vi "RX example.vi"() -> ()   [LabVIEW 2010]
uses:
  HackRF_Read_Complex.vi
  <vilib>/Analysis/NI_AALPro.lvlib
  <vilib>/Analysis/2dsp.llb/Complex FFT.vi
panel:
  out "Waveform Graph":dbl[](graph)
  in  "CarrierFreqHz":dbl(slide)=90658509.45494995 scale=86000000.0..110000000.0 scale format="%#_6p"
  in  "AMPEnable":bool
  in  "VGAGainDb":dbl=40.0 min=0.0 max=62.0 step=2.0
  in  "LNAGainDb":dbl=24.0 min=0.0 max=40.0 step=8.0
  in  "stop":bool
  in  "SampleFreqHz":dbl=4500000.0 format="%#_6p"
  in  "FilterBandwidthHz":dbl=3000000.0 format="%#_6p"
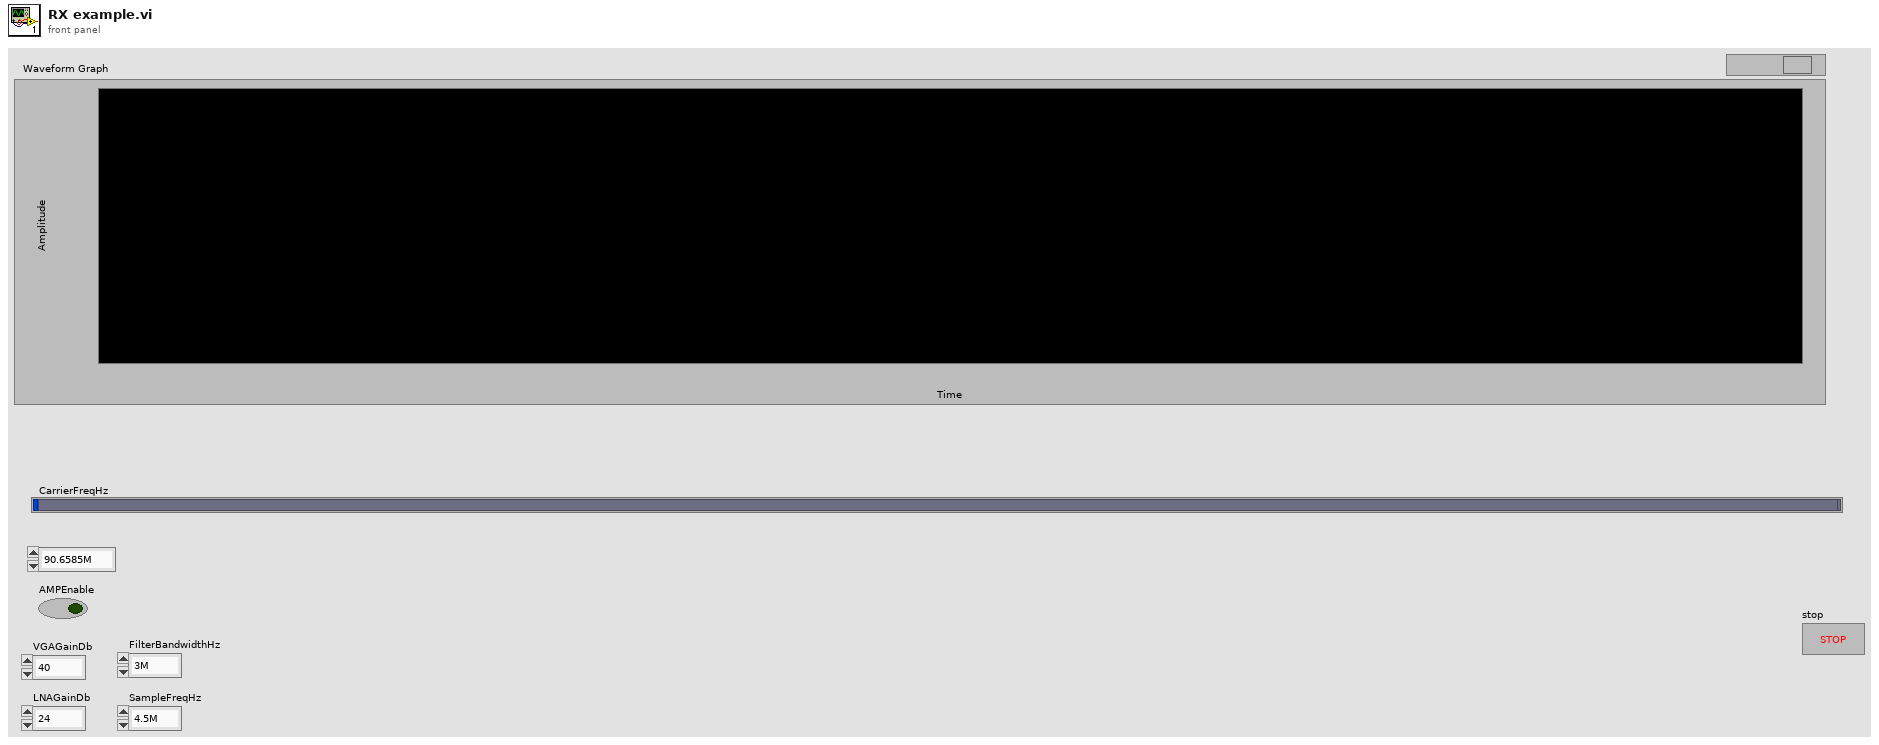
[diagram p1: front panel]
types:
  T1 = typedef "HackRF_Ref.ctl" = cluster{".net":refnum<k24>, "HackrfDeviceList":refnum<k24>[], "OpenDevice":refnum<k24>, "StartRX":refnum<k24>, "CarrierFreqHz":dbl, "SampleFreqHz":dbl, "FilterBandwidthHz":dbl, "AMPEnable":bool, "LNAGainDb":dbl, "VGAGainDb":dbl, "StartTx":refnum<k24>}
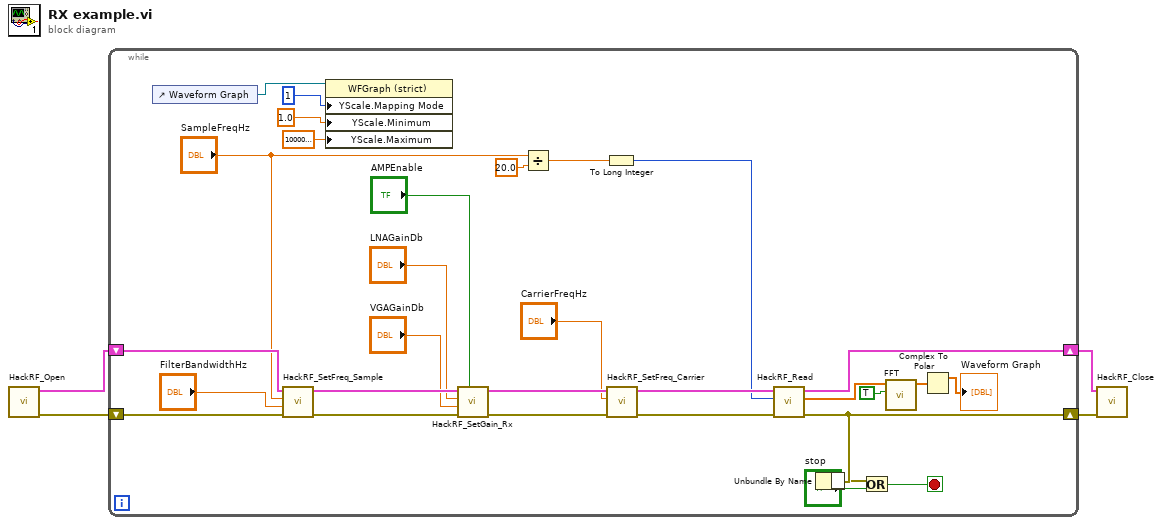
[diagram p0: block diagram]
diagram:
  n1 = call "HackRF_Open.vi"() -> ("error out"=w3:errorcluster, "Cluster"=w4:T1)  [unwired: 10 in]
  n2 = while {
    shift-right: [w18] -> w2
    shift-left: w4 -> [w34]
    shift-right: [w13] -> w1
    shift-left: w3 -> [w33]
    stop <- w11 stop-if-true
    n3 = control-ref of="Waveform Graph"() -> (w9:refnum<vi>)
    n4 = call "HackRF_SetFreq_Sample.vi"("error in (no error)"=w33, "FilterBandwidthHz"="FilterBandwidthHz", "SampleFreqHz"="SampleFreqHz", "HackRF in"=w34) -> ("error out"=w30:errorcluster, "HackRF out"=w31:T1)  [unwired: 6 in]
    n5 = property class="WFGraph (strict)"(reference=w9, "YScale.Mapping Mode"=u8 1 ("Y Scale.Mapping Mode"), "YScale.Minimum"=1.0 ("Y Scale.Range:Minimum"), "YScale.Maximum"=100000000.0 ("Y Scale.Range:Maximum")) -> ()  [unwired: 1 in, 2 out]
    n6 = call "HackRF_SetGain_Rx.vi"("AMPEnable"="AMPEnable", "error in (no error)"=w30, "VGAGainDb"="VGAGainDb", "LNAGainDb"="LNAGainDb", "HackRF in"=w31) -> ("error out"=w24:errorcluster, "HackRF out"=w27:T1)  [unwired: 5 in]
    n7 = Divide(x="SampleFreqHz", y=20.0) -> (x/y=w22:dbl)
    n8 = To Long Integer(number=w22) -> (32bit integer=w20:i32)
    n9 = call "HackRF_SetFreq_Carrier.vi"("error in (no error)"=w24, "CarrierFreqHz"="CarrierFreqHz", "HackRF_In"=w27) -> ("error out"=w19:errorcluster, "HackRF_Out"=w23:T1)  [unwired: 7 in]
    n10 = call-poly "HackRF_Read.vi"("error in (no error)"=w19, "count"=w20, "HackRF"=w23) -> ("error out"=w13:errorcluster, "Data"=w15:cdb[], "HackRF"=w18:T1)  [unwired: 6 in]
    n11 = Or(y="stop") -> (x=w5:errorcluster, x .or. y?=w11:bool)
    n12 = Unbundle By Name(w13, w5) -> ()
    n13 = call-poly <vilib>:"FFT.vi"("shift?"=TRUE, "X"=w15) -> ("FFT {X}"=w14:cdb[])  [unwired: 8 in, 1 out]
    n14 = Complex To Polar(r * e^(i*theta)=w14) -> (r=→"Waveform Graph":dbl[])  [unwired: 1 out]
  }
  n15 = call "HackRF_Close.vi"("error in (no error)"=w1, "Cluster in"=w2) -> ()  [unwired: 8 in, 2 out]
